vi "DB - [Execute].[ReportList].vi"(0 "connection reference":T6, 1 "DB Connection":T7={"Open"=TRUE, "Close"=TRUE}, 2 "?":T3=enum."INSERT INTO [Execute].[ReportList] ", 3 "AND <AND_CONDITION>":string, 5 "[ReportGenerateFail]":bool, 7 "[ReportRunNo]":string, 9 "Transaction":T5, 11 "error in (no error)":errorcluster, 12 "ReportList Cluster":T2, 13 "Logon":T4, 14 "Search Cluster":T1) -> (4 "connection reference":T6, 6 "data":string[][](array[string]), 8 "[ReportRunNo]":string, 15 "SUMMARY":errorcluster)   [LabVIEW 2013]
uses:
  <vilib>/addons/database/Connection.llb/Conn ObjectReference.ctl
  Controls/DB - OpenClose.ctl
  Controls/Transaction Cluster.ctl
  Controls/DB - Logon Info.ctl
  Controls/DB - Execute ReportList Enum.ctl
  Controls/Report List Cluster.ctl
  Controls/Global SRTRS.vi
  <vilib>/addons/database/Connection.llb/DB Tools Open Connec (String).vi
  <vilib>/addons/database/Connection.llb/Conn Execute.vi
  <vilib>/addons/database/Recordset.llb/Rec Fetch String Data (R).vi
  <vilib>/addons/database/Recordset.llb/Rec Destroy - Connection.vi
  <vilib>/addons/database/Recordset.llb/Rec Fetch Recordset Data (R).vi
  <vilib>/addons/database/_DB Variant To Data/Database Variant To Data.xnode
  <vilib>/addons/database/NI_Database_API.lvlib
panel:
  out "Error Out":errorcluster
  out "SQL Statement":string
  in  "DB.Schema.Table \nSRTRS.Execute.ReportList":string="SRTRS.Execute.ReportList"
  in  "DB.Schema.Table\nSRTRS.Execute.TransactionReport":string="SRTRS.Execute.TransactionReport"
  out "Connection Information":T8={"Connection "="SQL Server 32bit HPEnvy", "Username"="admin", "Password"="admin123"}
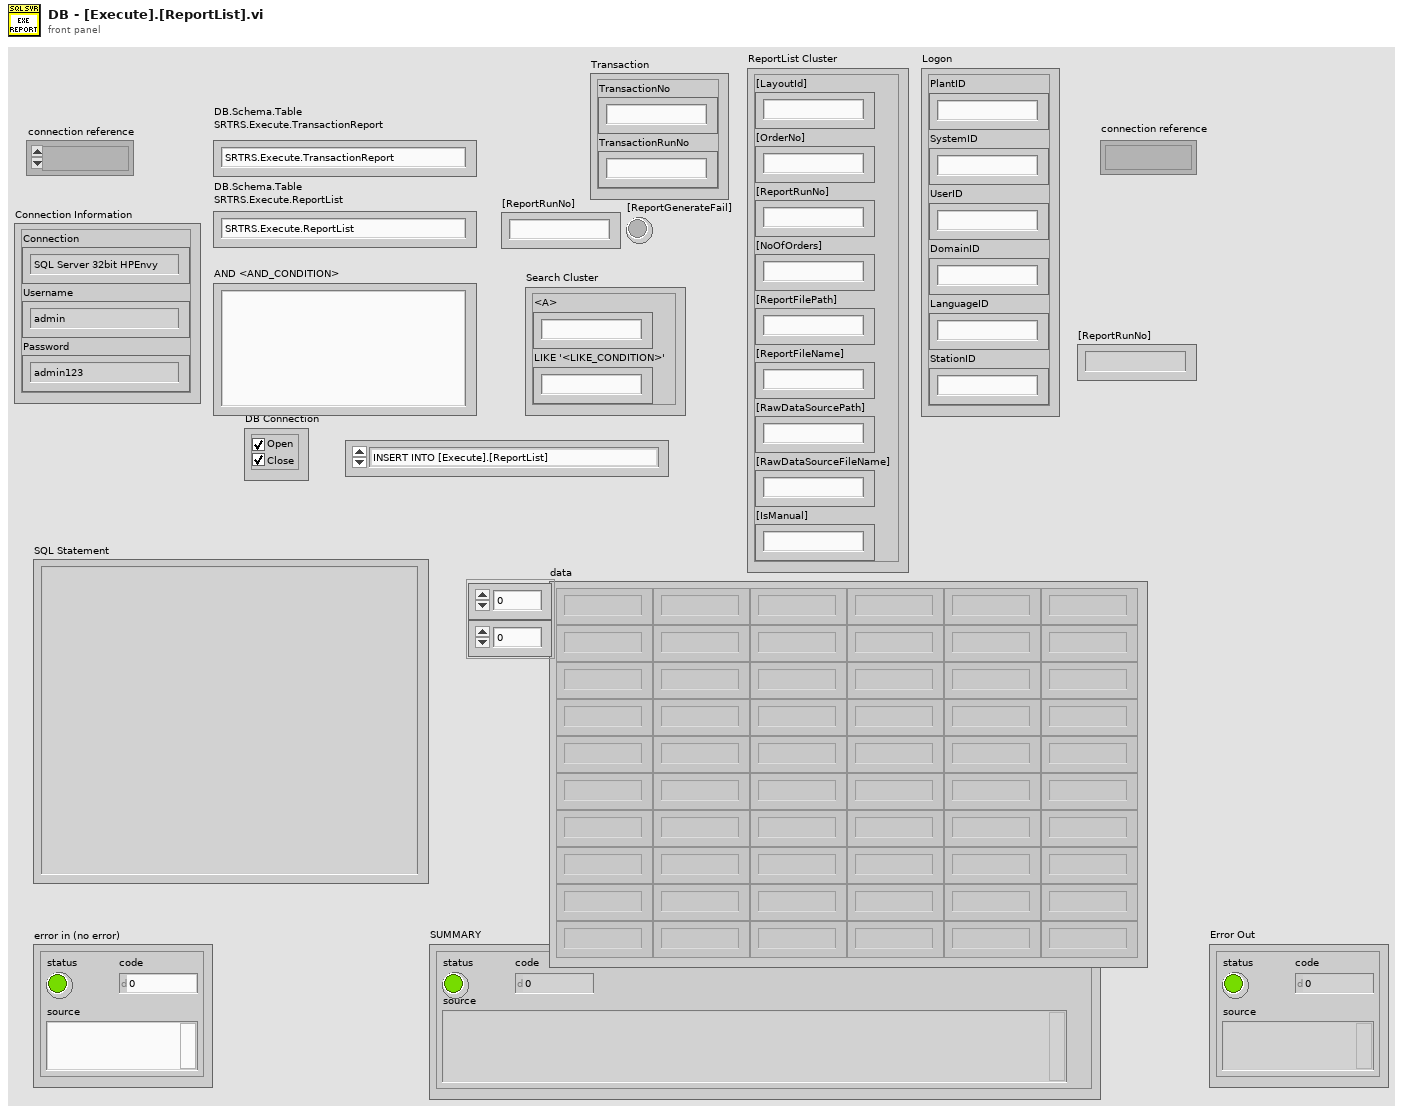
[diagram p1: front panel]
types:
  T1 = cluster{"<A>":string, "LIKE '<LIKE_CONDITION>'":string}
  T2 = typedef "Report List Cluster.ctl" = cluster{"[LayoutId]":string, "[OrderNo]":string, "[ReportRunNo]":string, "[NoOfOrders]":string, "[ReportFilePath]":string, "[ReportFileName]":string, "[RawDataSourcePath]":string, "[RawDataSourceFileName]":string, "[IsManual]":string}
  T3 = typedef "DB - Execute ReportList Enum.ctl" = enum16{"INSERT INTO [Execute].[TransactionReport]", "UPDATE [Execute].[TransactionReport]", "INSERT INTO [Execute].[ReportList] ", "SELECT [TransactionNo] OR [OrderNo]", "SELECT [TransactionNo],* OR [OrderNo],*", "SELECT [ReportFileName]"}
  T4 = typedef "DB - Logon Info.ctl" = cluster{"PlantID":string, "SystemID":string, "UserID":string, "DomainID":string, "LanguageID":string, "StationID":string}
  T5 = typedef "Transaction Cluster.ctl" = cluster{"TransactionNo":string, "TransactionRunNo":string}
  T6 = typedef "NI_Database_API.lvlib/Conn ObjectReference.ctl" = refnum<k1>
  T7 = typedef "DB - OpenClose.ctl" = cluster{"Open":bool, "Close":bool}
  T8 = cluster{"Connection ":string, "Username":string, "Password":string}
  T9 = typedef "Enum - InteractiveMode-SubVIMode.ctl" = enum16{"Interactive", "subVI Mode"}
  T10 = typedef "DB - DB.Schema.Table.ctl" = cluster{"DB":string, "Schema":string, "Table":string}
  T11 = typedef "Connection Information Cluster.ctl" = cluster{"Connection ":string, "Username":string, "Password":string}
  T12 = typedef "NI_Database_API.lvlib/Rec ObjectReference.ctl" = refnum<k1>
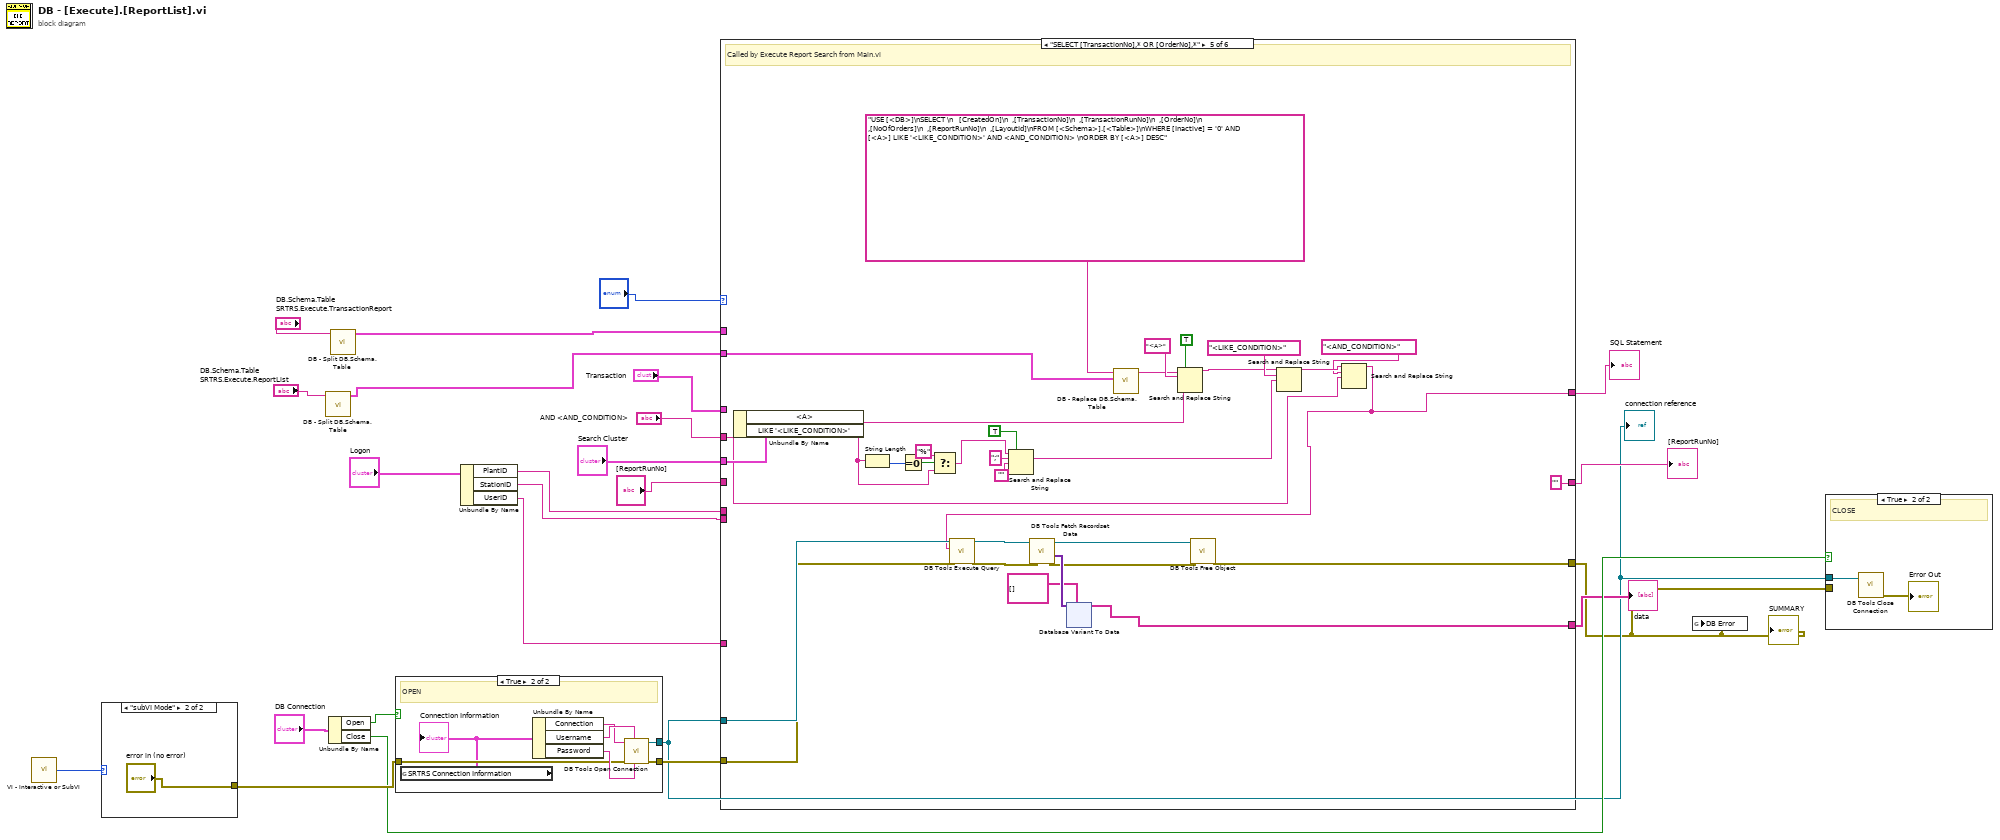
[diagram p0: block diagram]
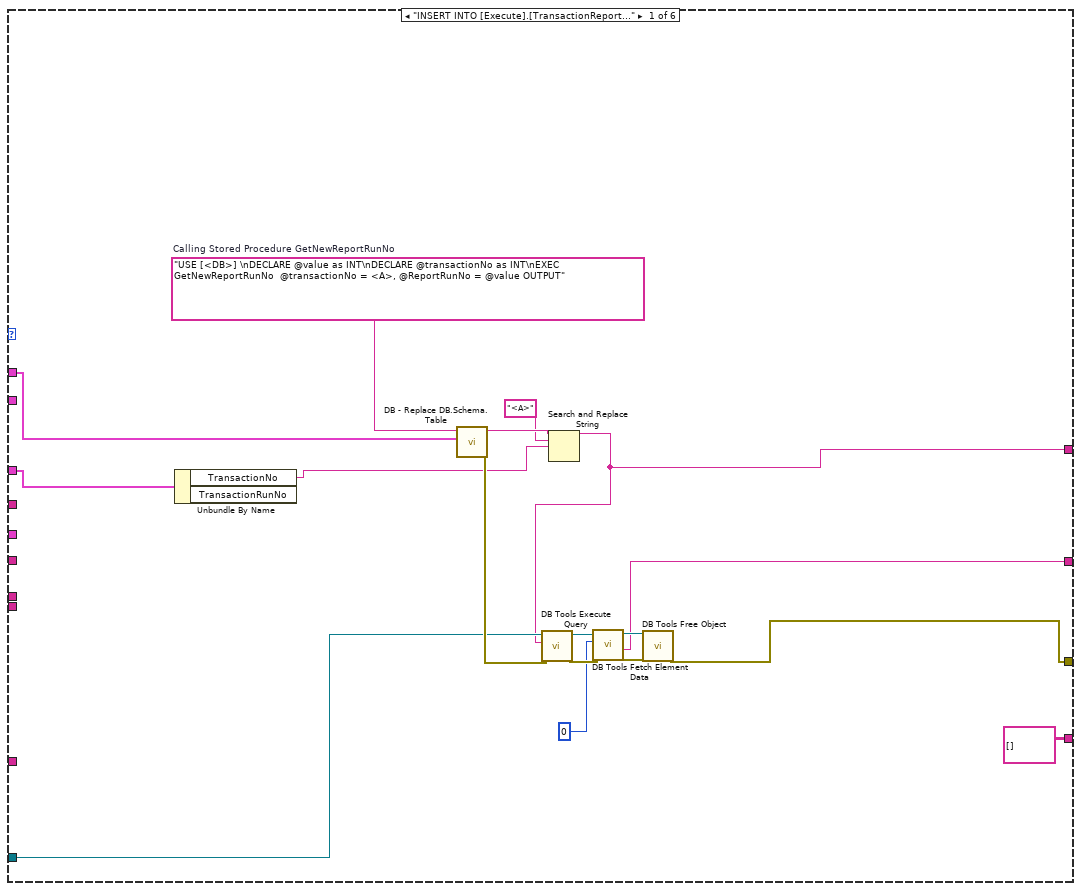
[diagram p2: hidden frame]
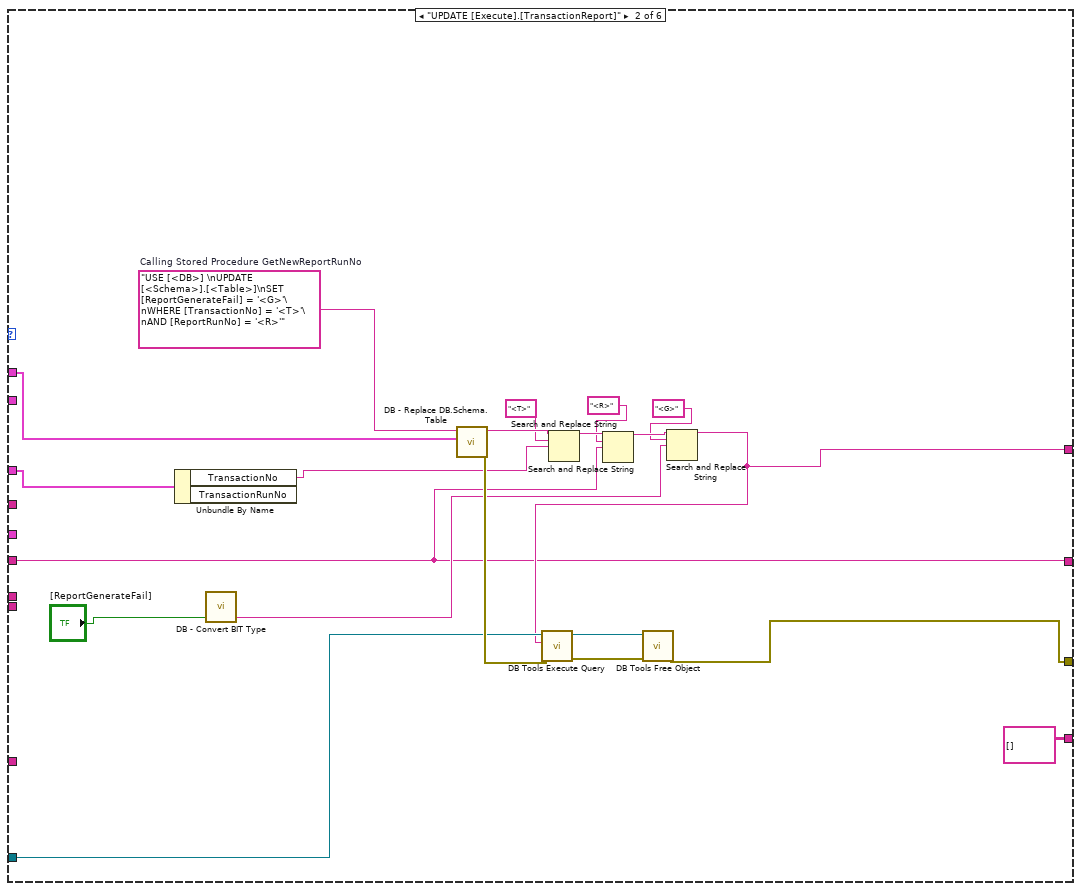
[diagram p3: hidden frame]
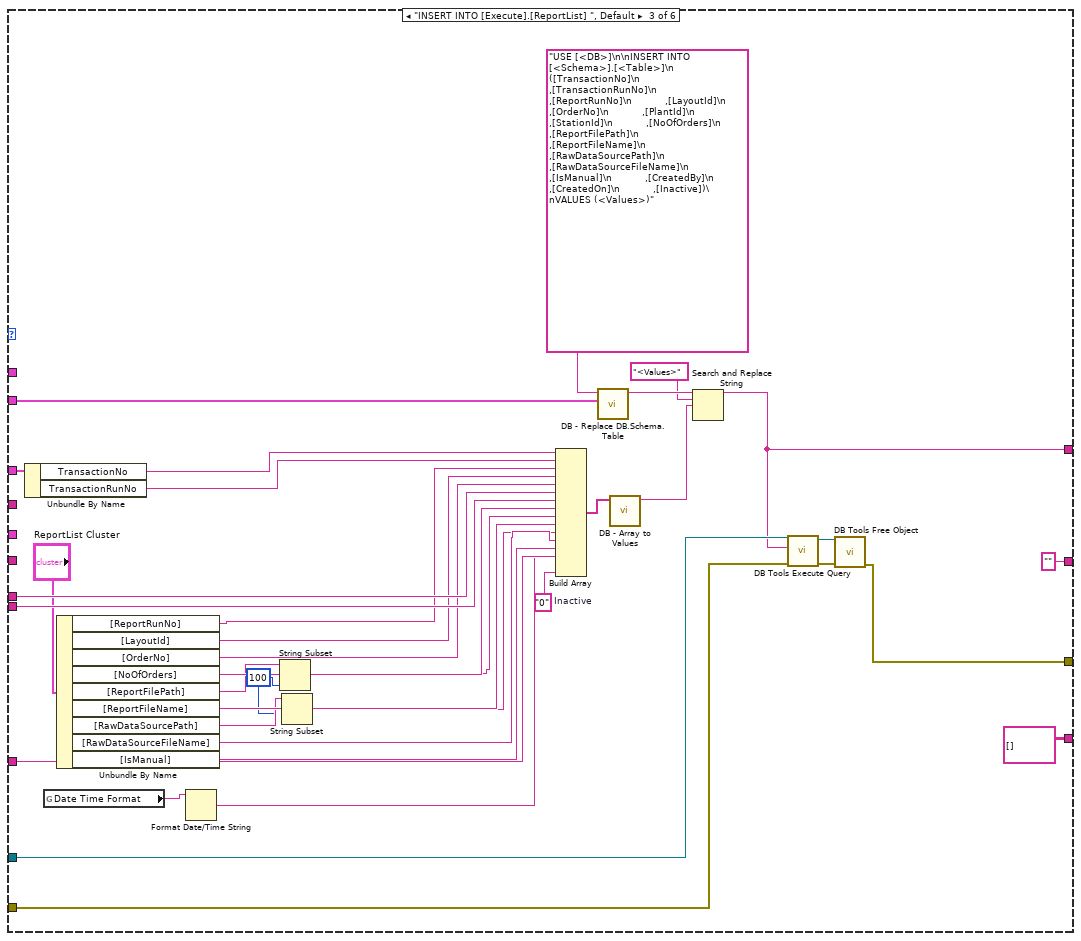
[diagram p4: hidden frame]
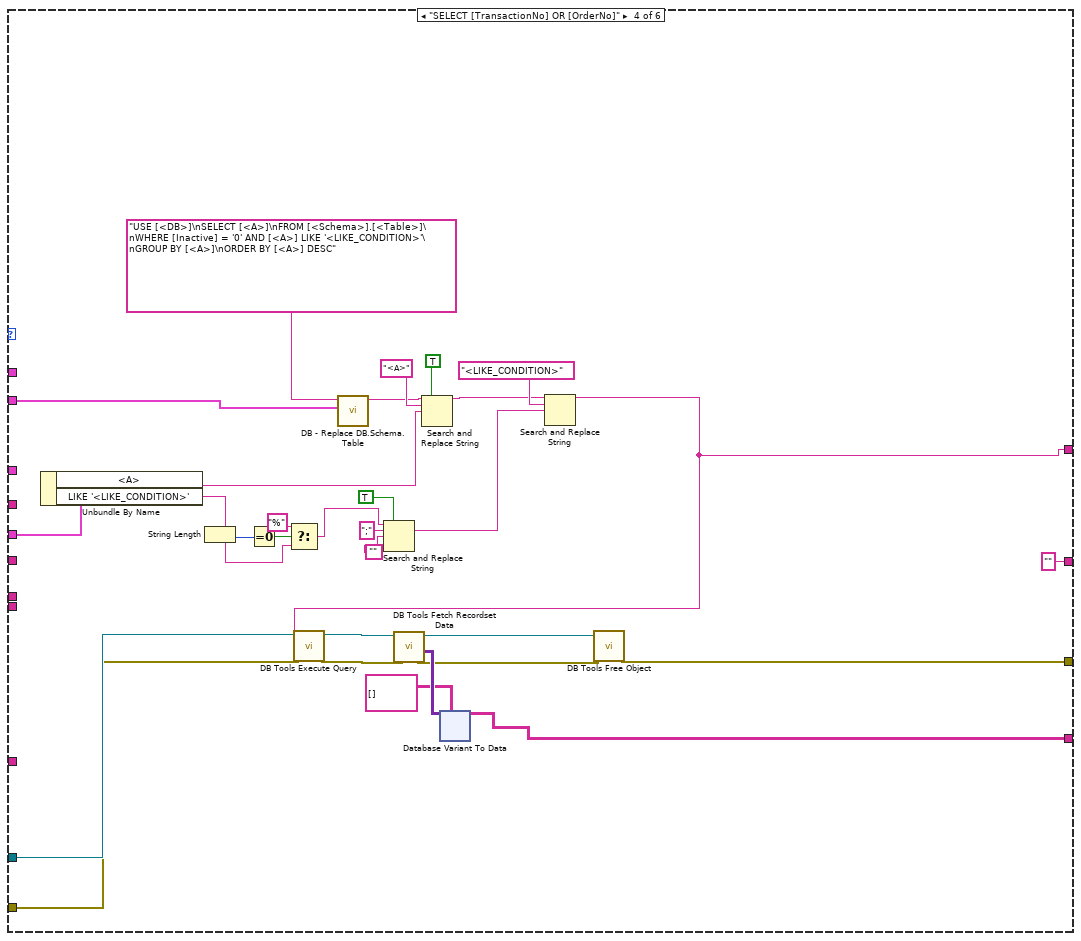
[diagram p5: hidden frame]
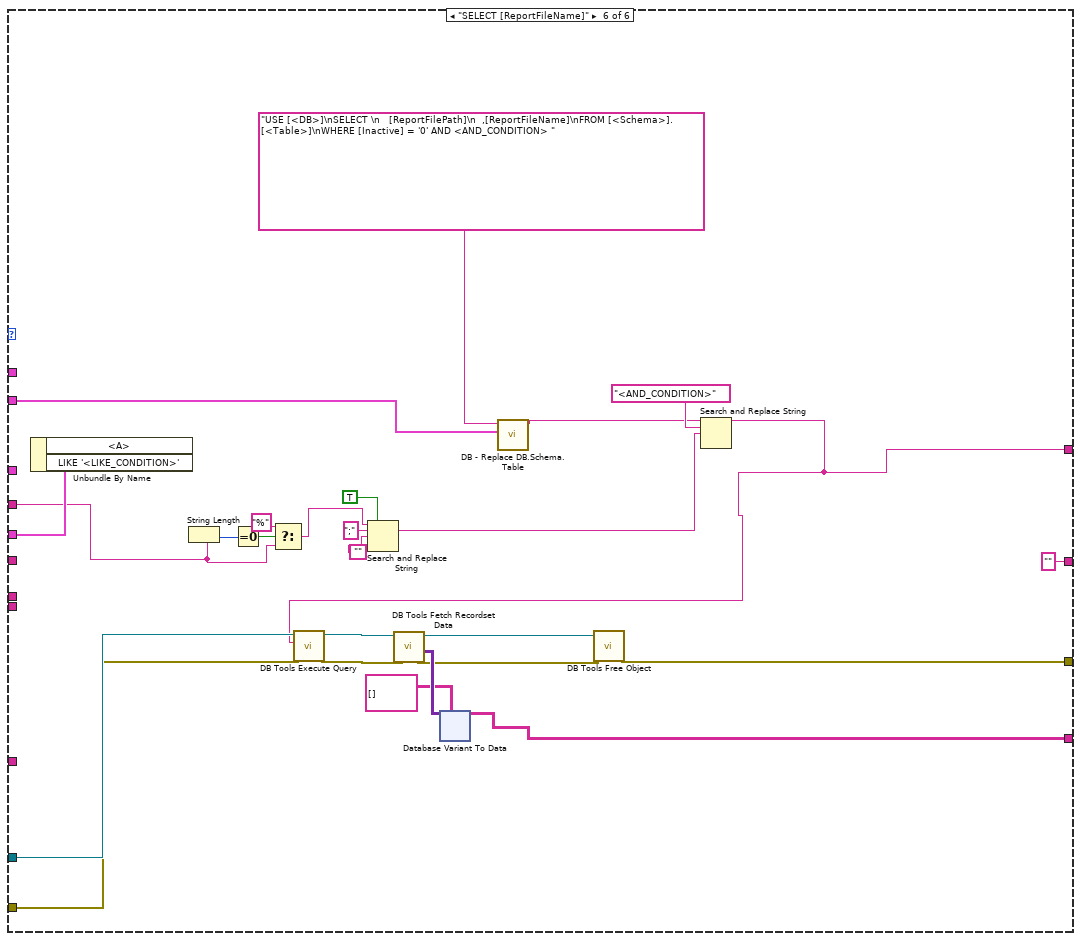
[diagram p6: hidden frame]
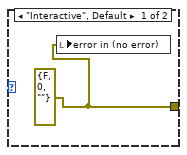
[diagram p8: hidden frame]
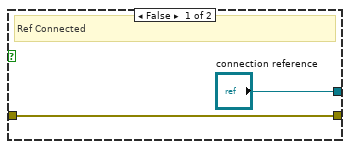
[diagram p9: hidden frame]
diagram:
  n1 = call "VI - Interactive or SubVI.vi"() -> ("Mode"=w22:T9)  [unwired: 5 in]
  n2 = case shown="\"subVI Mode\"" w22 {
    tunnel: [w25 "error in (no error)"] -> w21
    frame "Interactive", Default {
      w25 = errorcluster {"status"=FALSE, "code"=0, "source"=""} ("error in (no error)")
      n3 = local write "error in (no error)"(w25) -> ()
    }
    frame "subVI Mode" {
    }
  }
  n4 = call "DB - Split DB.Schema.Table.vi"("DB.Schema.Table"="DB.Schema.Table \nSRTRS.Execute.ReportList") -> ("DB.Schema.Table"=w11:T10)  [unwired: 10 in]
  n5 = Unbundle By Name("DB Connection") -> ("Open"=w23:bool, "Close"=w19:bool)
  n6 = call "DB - Split DB.Schema.Table.vi"("DB.Schema.Table"="DB.Schema.Table\nSRTRS.Execute.TransactionReport") -> ("DB.Schema.Table"=w16:T10)  [unwired: 10 in]
  n7 = case shown="True" w23 {
    tunnel: ["connection reference" w32] -> w12
    tunnel: w21 -> [w27 w31]
    tunnel: [w27 w30] -> w20
    frame False {
      # "Ref Connected"
    }
    frame True {
      # "OPEN"
      n8 = global read "Global SRTRS.vi" "SRTRS Connection Information"() -> (w29:T11)
      "Connection Information" <- w29
      n9 = Unbundle By Name(w29) -> ("Connection"=w34:string, "Username"=w35:string, "Password"=w33:string)
      n10 = call-poly <vilib>:"DB Tools Open Connection.vi"("password"=w33, "userID"=w35, "error in (no error)"=w31, "connection information"=w34) -> ("error out"=w30:errorcluster, "connection reference"=w32:T6)  [unwired: 4 in]
    }
  }
  "connection reference" <- w12
  n11 = Unbundle By Name("Logon") -> ("PlantID"=w9:string, "StationID"=w8:string, "UserID"=w7:string)
  n12 = case shown="\"SELECT [TransactionNo],* OR [OrderNo],*\"" "?" {
    tunnel: w12 -> [w49 w69 w90 w132 w209 w279]
    tunnel: w20 -> [_ _ w89 w131 w208 w278]
    tunnel: [w48 w68 w81 w130 w207 w277] -> w3
    tunnel: w16 -> [w50 w70 _ _ _ _]
    tunnel: w9 -> [_ _ w101 _ _ _]
    tunnel: "Transaction" -> [w47 w67 w104 _ _ _]
    tunnel: [string[][] [] ("data") string[][] [] ("data") string[][] [] ("data") w128 w204 w274] -> w14
    tunnel: [w38 w55 "" ("data") "" ("data") "" ("data") "" ("data")] -> w13
    tunnel: w11 -> [_ _ w108 w126 w202 w272]
    tunnel: w8 -> [_ _ w100 _ _ _]
    tunnel: w7 -> [_ _ w99 _ _ _]
    tunnel: [w37 w60 w84 w109 w185 w261] -> w6
    tunnel: "Search Cluster" -> [_ _ _ w117 w191 w263]
    tunnel: "AND <AND_CONDITION>" -> [_ _ _ _ w183 w260]
    tunnel: "[ReportRunNo]" -> [_ w55 _ _ _ _]
    frame "INSERT INTO [Execute].[TransactionReport]" {
      w51 = "USE [<DB>] \nDECLARE @value as INT\nDECLARE @transactionNo as INT\nEXEC GetNewReportRunNo  @transactionNo = <A>, @ReportRunNo = @value OUTPUT"  # Calling Stored Procedure GetNewReportRunNo
      n13 = Unbundle By Name(w47) -> ("TransactionNo"=w44:string)  [unwired: 1 out]
      n14 = call "DB - Replace DB.Schema.Table.vi"("DB.Schema.Table"=w50, "string in"=w51) -> ("error out"=w52:errorcluster, "string out"=w46:string)  [unwired: 8 in]
      n15 = Search and Replace String(input string=w46, search string="<A>", replace string=w44) -> (result string=w37:string)  [unwired: 5 in, 3 out]
      n16 = call-poly <vilib>:"DB Tools Execute Query.vi"("error in (no error)"=w52, "SQL query"=w37, "connection reference"=w49) -> ("error out"=w43:errorcluster, "recordset reference"=w42:T12)  [unwired: 5 in]
      n17 = call-poly <vilib>:"DB Tools Fetch Element Data.vi"("error in (no error)"=w43, "column index"=0, "recordset reference"=w42) -> ("error out"=w41:errorcluster, "data"=w38:string, "recordset reference out"=w40:T12)  [unwired: 4 in]
      n18 = call-poly <vilib>:"DB Tools Free Object.vi"("error in (no error)"=w41, "recordset reference"=w40) -> ("error out"=w48:errorcluster)  [unwired: 8 in, 1 out]
    }
    frame "UPDATE [Execute].[TransactionReport]" {
      w71 = "USE [<DB>] \nUPDATE [<Schema>].[<Table>]\nSET [ReportGenerateFail] = '<G>'\nWHERE [TransactionNo] = '<T>'\nAND [ReportRunNo] = '<R>'"  # Calling Stored Procedure GetNewReportRunNo
      n19 = Unbundle By Name(w67) -> ("TransactionNo"=w64:string)  [unwired: 1 out]
      n20 = call "DB - Convert BIT Type.vi"("Boolean"="[ReportGenerateFail]") -> ("BIT (eg Inactive)"=w56:string)  [unwired: 2 in, 2 out]
      n21 = call "DB - Replace DB.Schema.Table.vi"("DB.Schema.Table"=w70, "string in"=w71) -> ("error out"=w72:errorcluster, "string out"=w66:string)  [unwired: 8 in]
      n22 = Search and Replace String(input string=w66, search string="<T>", replace string=w64) -> (result string=w62:string)  [unwired: 5 in, 3 out]
      n23 = Search and Replace String(input string=w62, search string="<R>", replace string=w55) -> (result string=w61:string)  [unwired: 5 in, 3 out]
      n24 = Search and Replace String(input string=w61, search string="<G>", replace string=w56) -> (result string=w60:string)  [unwired: 5 in, 3 out]
      n25 = call-poly <vilib>:"DB Tools Execute Query.vi"("error in (no error)"=w72, "SQL query"=w60, "connection reference"=w69) -> ("error out"=w54:errorcluster, "recordset reference"=w53:T12)  [unwired: 5 in]
      n26 = call-poly <vilib>:"DB Tools Free Object.vi"("error in (no error)"=w54, "recordset reference"=w53) -> ("error out"=w68:errorcluster)  [unwired: 8 in, 1 out]
    }
    frame "INSERT INTO [Execute].[ReportList] ", Default {
      w75 = 100 ("length (rest)")
      w91 = "0"  # Inactive
      n27 = Unbundle By Name(w104) -> ("TransactionNo"=w103:string, "TransactionRunNo"=w102:string)
      n28 = global read "Global SRTRS.vi" "Date Time Format"() -> (w92:string)
      n29 = Unbundle By Name("ReportList Cluster") -> ("[ReportRunNo]"=w73:string, "[LayoutId]"=w97:string, "[OrderNo]"=w96:string, "[NoOfOrders]"=w95:string, "[ReportFilePath]"=w78:string, "[ReportFileName]"=w94:string, "[RawDataSourcePath]"=w76:string, "[RawDataSourceFileName]"=w79:string, "[IsManual]"=w93:string)
      n30 = Format Date/Time String(time format string (%c)=w92) -> (date/time string=w80:string)  [unwired: 2 in]
      n31 = String Subset(string=w78, length (rest)=w75) -> (substring=w77:string)  [unwired: 1 in]
      n32 = String Subset(string=w76, offset (0)=w75) -> (substring=w74:string)  [unwired: 1 in]
      n33 = Build Array(w103, w102, w73, w97, w96, w101, w100, w95, w77, w94, w74, w79, w93, w99, w80, w91) -> (w105:string[])
      n34 = call "DB - Replace DB.Schema.Table.vi"("DB.Schema.Table"=w108, "string in"="USE [<DB>]\n\nINSERT INTO [<Schema>].[<Table>]\n           ([TransactionNo]\n           ,[TransactionRunNo]\n           ,[ReportRunNo]\n           ,[LayoutId]\n           ,[OrderNo]\n           ,[PlantId]\n           ,[StationId]\n           ,[NoOfOrders]\n           ,[ReportFilePath]\n           ,[ReportFileName]\n           ,[RawDataSourcePath]\n           ,[RawDataSourceFileName]\n           ,[IsManual]\n           ,[CreatedBy]\n           ,[CreatedOn]\n           ,[Inactive])\nVALUES (<Values>)") -> ("string out"=w106:string)  [unwired: 8 in, 1 out]
      n35 = call "DB - Array to Values.vi"("Array (0xFFFE autodetect)"=w105) -> ("<Values>"=w82:string)  [unwired: 10 in]
      n36 = Search and Replace String(input string=w106, search string="<Values>" ("replace string (\"\")"), replace string=w82) -> (result string=w84:string)  [unwired: 5 in, 3 out]
      n37 = call-poly <vilib>:"DB Tools Execute Query.vi"("error in (no error)"=w89, "SQL query"=w84, "connection reference"=w90) -> ("error out"=w88:errorcluster, "recordset reference"=w87:T12)  [unwired: 5 in]
      n38 = call-poly <vilib>:"DB Tools Free Object.vi"("error in (no error)"=w88, "recordset reference"=w87) -> ("error out"=w81:errorcluster)  [unwired: 8 in, 1 out]
    }
    frame "SELECT [TransactionNo] OR [OrderNo]" {
      n39 = Unbundle By Name(w117) -> ("<A>"=w111:string, "LIKE '<LIKE_CONDITION>'"=w118:string)
      n40 = String Length(string=w118) -> (length=w124:i32)
      n41 = Equal To 0?(x=w124) -> (x = 0?=w125:bool)
      n42 = Select(t="%", s=w125, f=w118) -> (s? t:f=w122:string)
      n43 = call "DB - Replace DB.Schema.Table.vi"("DB.Schema.Table"=w126, "string in"="USE [<DB>]\nSELECT [<A>]\nFROM [<Schema>].[<Table>]\nWHERE [Inactive] = '0' AND [<A>] LIKE '<LIKE_CONDITION>'\nGROUP BY [<A>]\nORDER BY [<A>] DESC") -> ("string out"=w112:string)  [unwired: 8 in, 1 out]
      n44 = Search and Replace String(replace all?=TRUE ("replace all? (F)"), input string=w122, search string=";", replace string="") -> (result string=w110:string)  [unwired: 4 in, 3 out]
      n45 = Search and Replace String(replace all?=TRUE ("replace all? (F)"), input string=w112, search string="<A>", replace string=w111) -> (result string=w113:string)  [unwired: 4 in, 3 out]
      n46 = Search and Replace String(input string=w113, search string="<LIKE_CONDITION>", replace string=w110) -> (result string=w109:string)  [unwired: 5 in, 3 out]
      n47 = call-poly <vilib>:"DB Tools Execute Query.vi"("error in (no error)"=w131, "SQL query"=w109, "connection reference"=w132) -> ("error out"=w138:errorcluster, "recordset reference"=w137:T12)  [unwired: 5 in]
      n48 = call-poly <vilib>:"DB Tools Fetch Recordset Data.vi"("error in (no error)"=w138, "recordset reference"=w137) -> ("error out"=w133:errorcluster, "recordset data"=w136:variant[][], "recordset reference out"=w134:T12)  [unwired: 3 in]
      n49 = xnode "Database Variant To Data"("database variant"=w136, "type"=string[][] []) -> ("data"=w128:string[][])  [unwired: 1 in, 1 out]
      n50 = call-poly <vilib>:"DB Tools Free Object.vi"("error in (no error)"=w133, "recordset reference"=w134) -> ("error out"=w130:errorcluster)  [unwired: 8 in, 1 out]
    }
    frame "SELECT [TransactionNo],* OR [OrderNo],*" {
      # "Called by Execute Report Search from Main.vi"
      n51 = Unbundle By Name(w191) -> ("<A>"=w190:string, "LIKE '<LIKE_CONDITION>'"=w189:string)
      n52 = String Length(string=w189) -> (length=w200:i32)
      n53 = Equal To 0?(x=w200) -> (x = 0?=w201:bool)
      n54 = Select(t="%", s=w201, f=w189) -> (s? t:f=w198:string)
      n55 = Search and Replace String(replace all?=TRUE ("replace all? (F)"), input string=w198, search string=";", replace string="") -> (result string=w193:string)  [unwired: 4 in, 3 out]
      n56 = call "DB - Replace DB.Schema.Table.vi"("DB.Schema.Table"=w202, "string in"="USE [<DB>]\nSELECT \n   [CreatedOn]\n  ,[TransactionNo]\n  ,[TransactionRunNo]\n  ,[OrderNo]\n  ,[NoOfOrders]\n  ,[ReportRunNo]\n  ,[LayoutId]\nFROM [<Schema>].[<Table>]\nWHERE [Inactive] = '0' AND [<A>] LIKE '<LIKE_CONDITION>' AND <AND_CONDITION> \nORDER BY [<A>] DESC") -> ("string out"=w188:string)  [unwired: 8 in, 1 out]
      n57 = Search and Replace String(replace all?=TRUE ("replace all? (F)"), input string=w188, search string="<A>", replace string=w190) -> (result string=w187:string)  [unwired: 4 in, 3 out]
      n58 = Search and Replace String(input string=w187, search string="<LIKE_CONDITION>", replace string=w193) -> (result string=w186:string)  [unwired: 5 in, 3 out]
      n59 = Search and Replace String(input string=w186, search string="<AND_CONDITION>", replace string=w183) -> (result string=w185:string)  [unwired: 5 in, 3 out]
      n60 = call-poly <vilib>:"DB Tools Execute Query.vi"("error in (no error)"=w208, "SQL query"=w185, "connection reference"=w209) -> ("error out"=w215:errorcluster, "recordset reference"=w214:T12)  [unwired: 5 in]
      n61 = call-poly <vilib>:"DB Tools Fetch Recordset Data.vi"("error in (no error)"=w215, "recordset reference"=w214) -> ("error out"=w210:errorcluster, "recordset data"=w213:variant[][], "recordset reference out"=w211:T12)  [unwired: 3 in]
      n62 = xnode "Database Variant To Data"("database variant"=w213, "type"=string[][] []) -> ("data"=w204:string[][])  [unwired: 1 in, 1 out]
      n63 = call-poly <vilib>:"DB Tools Free Object.vi"("error in (no error)"=w210, "recordset reference"=w211) -> ("error out"=w207:errorcluster)  [unwired: 8 in, 1 out]
    }
    frame "SELECT [ReportFileName]" {
      n64 = Unbundle By Name(w263) -> ()  [unwired: 2 out]
      n65 = String Length(string=w260) -> (length=w270:i32)
      n66 = Equal To 0?(x=w270) -> (x = 0?=w271:bool)
      n67 = Select(t="%", s=w271, f=w260) -> (s? t:f=w268:string)
      n68 = Search and Replace String(replace all?=TRUE ("replace all? (F)"), input string=w268, search string=";", replace string="") -> (result string=w264:string)  [unwired: 4 in, 3 out]
      n69 = call "DB - Replace DB.Schema.Table.vi"("DB.Schema.Table"=w272, "string in"="USE [<DB>]\nSELECT \n   [ReportFilePath]\n  ,[ReportFileName]\nFROM [<Schema>].[<Table>]\nWHERE [Inactive] = '0' AND <AND_CONDITION> ") -> ("string out"=w262:string)  [unwired: 8 in, 1 out]
      n70 = Search and Replace String(input string=w262, search string="<AND_CONDITION>", replace string=w264) -> (result string=w261:string)  [unwired: 5 in, 3 out]
      n71 = call-poly <vilib>:"DB Tools Execute Query.vi"("error in (no error)"=w278, "SQL query"=w261, "connection reference"=w279) -> ("error out"=w285:errorcluster, "recordset reference"=w284:T12)  [unwired: 5 in]
      n72 = call-poly <vilib>:"DB Tools Fetch Recordset Data.vi"("error in (no error)"=w285, "recordset reference"=w284) -> ("error out"=w280:errorcluster, "recordset data"=w283:variant[][], "recordset reference out"=w281:T12)  [unwired: 3 in]
      n73 = xnode "Database Variant To Data"("database variant"=w283, "type"=string[][] []) -> ("data"=w274:string[][])  [unwired: 1 in, 1 out]
      n74 = call-poly <vilib>:"DB Tools Free Object.vi"("error in (no error)"=w280, "recordset reference"=w281) -> ("error out"=w277:errorcluster)  [unwired: 8 in, 1 out]
    }
  }
  "SUMMARY" <- w3
  "data" <- w14
  "[ReportRunNo]" <- w13
  "SQL Statement" <- w6
  n75 = global write "Global SRTRS.vi" "DB Error"(w3) -> ()
  n76 = case shown="True" w19 {
    tunnel: w12 -> [_ w331]
    tunnel: w3 -> [_ _]
    frame False {
      # "Ref Connected"
    }
    frame True {
      # "CLOSE"
      n77 = call <vilib>:"DB Tools Close Connection.vi"("connection reference"=w331) -> ("error out"=→"Error Out":errorcluster)  [unwired: 6 in]
    }
  }
